vi "get className.vi"(8 "error in (no error)":errorcluster, 11 "xceNode in":refnum<class "xceNode.lvclass">) -> (0 "error out":errorcluster, 2 "Class name":string, 3 "xceNode out":refnum<class "xceNode.lvclass">)   [LabVIEW 2013, in "xceNode.lvclass"]
doc: "Returns the name of the class instance."
uses:
  xceNode.lvclass
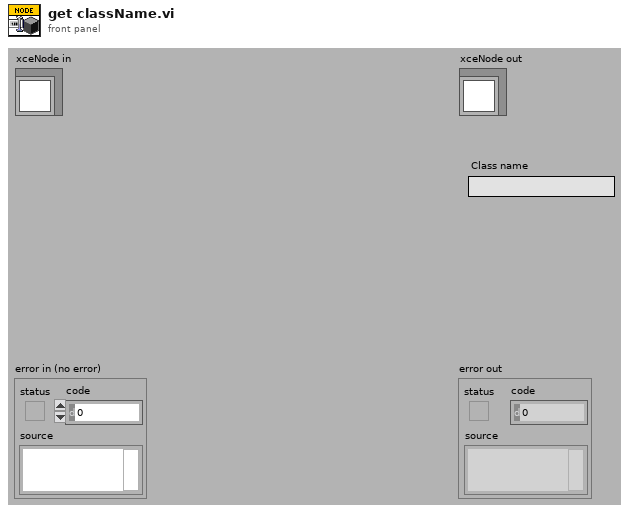
[diagram p1: front panel]
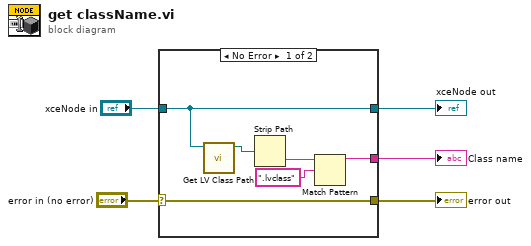
[diagram p0: block diagram]
diagram:
  n1 = case shown="No Error" "error in (no error)" {
    selector: "error in (no error)" -> [w11 w13]
    tunnel: [w11 w13] -> w4
    tunnel: [w10 w12] -> w2
    tunnel: "xceNode in" -> [w10 w12]
    tunnel: [w6 _] -> w1
    frame No Error {
      n2 = call <vilib>:"Get LV Class Path.vi"("object"=w10) -> ("class path"=w9:path)  [unwired: 9 in, 1 out]
      n3 = Strip Path(path=w9) -> (name=w8:string)  [unwired: 1 out]
      n4 = Match Pattern(string=w8, regular expression=".lvclass") -> (before substring=w6:string)  [unwired: 1 in, 3 out]
    }
    frame Error {
    }
  }
  "error out" <- w4
  "xceNode out" <- w2
  "Class name" <- w1
